vi "Is_acquisition_running.vi"(8 "error in (no error)":errorcluster, 11 ".NET Refnum in":refnum<k24>) -> (0 "error out":errorcluster, 3 "bValue":bool)   [LabVIEW 2021]
uses:
  C:/Program Files/Thorlabs/Scientific Imaging/ThorCam/uc480DotNet.dll
  Program Files/Thorlabs/Scientific Imaging/ThorCam/uc480DotNet.dll
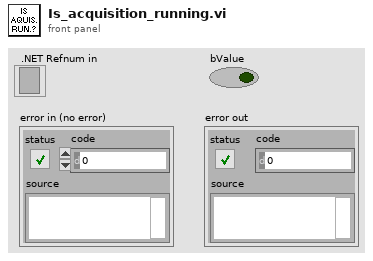
[diagram p1: front panel]
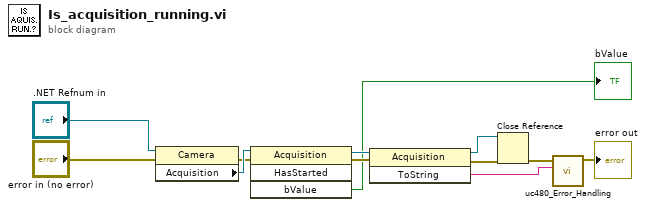
[diagram p0: block diagram]
diagram:
  n1 = property class="Camera"(reference=".NET Refnum in", error in="error in (no error)") -> (error out=w1:errorcluster, "Acquisition"=w2:refnum<k24>)  [unwired: 1 out]
  n2 = invoke class="Acquisition" method="HasStarted"(reference=w2, error in=w1) -> (reference out=w7:refnum<k24>, error out=w5:errorcluster, "bValue"=→"bValue":bool)  [unwired: 2 in, 1 out]
  n3 = invoke class="Acquisition" method="ToString"(reference=w7, error in=w5) -> (reference out=w12:refnum<k24>, error out=w10:errorcluster, "ToString"=w6:string)  [unwired: 1 in]
  n4 = Close Reference(reference=w12, error in (no error)=w10) -> (error out=w11:errorcluster)
  n5 = call "uc480_Error_Handling.vi"("Error String"=w6, "Error In"=w11) -> ("Error Out"=→"error out":errorcluster)  [unwired: 9 in]
